vi "uTTA_SetMaxMultiplier.vi"(8 "error in":errorcluster, 10 "Max Multiplier":u16, 11 "VISA Refnum in":refnum<visa-resource-name>) -> (0 "error out":errorcluster, 1 "SamplingSettings":T1, 2 "Received":string, 3 "VISA Refnum out":refnum<visa-resource-name>)   [LabVIEW 2021]
uses:
  uTTA_Controls/CTL_uTTA_SamplingSettings.ctl
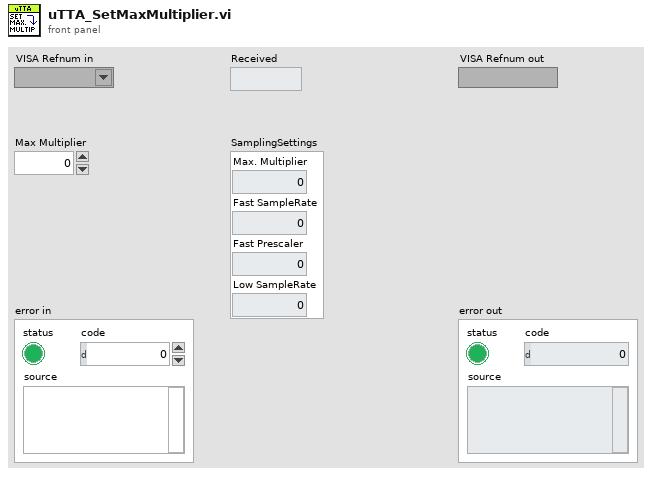
[diagram p1: front panel]
types:
  T1 = typedef "CTL_uTTA_SamplingSettings.ctl" = cluster{"Max. Multiplier":i32, "Fast SampleRate":i32, "Fast Prescaler":dbl, "Low SampleRate":dbl}
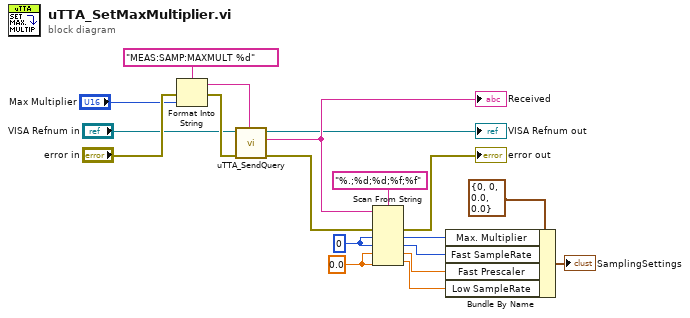
[diagram p0: block diagram]
diagram:
  w19 = 0.0 ("default value 1")
  w18 = 0 ("default value 1")
  n1 = Format Into String(format string="MEAS:SAMP:MAXMULT %d", error in="error in", "Max Multiplier") -> (resulting string=w11:string, error out=w13:errorcluster)  [unwired: 1 in]
  n2 = call "uTTA_SendQuery.vi"("Send String"=w11, "error in (no error)"=w13, "VISA Refnum in"="VISA Refnum in") -> ("error out"=w16:errorcluster, "Received"=w14:string, "VISA Refnum out"=→"VISA Refnum out":refnum<visa-resource-name>)  [unwired: 6 in]
  "Received" <- w14
  n3 = Scan From String(format string="%.;%d;%d;%f;%f", input string=w14, error in=w16, default 1=w18, default 2=w18, default 3=w19, default 4=w19) -> (error out=→"error out":errorcluster, output 1=w5:i32, output 2=w4:i32, output 3=w3:dbl, output 4=w2:dbl)  [unwired: 1 in, 2 out]
  n4 = Bundle By Name(cluster=T1 {"Max. Multiplier"=0, "Fast SampleRate"=0, "Fast Prescaler"=0.0, "Low SampleRate"=0.0} ("SamplingSettings"), "Max. Multiplier"=w5, "Fast SampleRate"=w4, "Fast Prescaler"=w3, "Low SampleRate"=w2) -> (→"SamplingSettings":T1)
